vi "Generate Error.vi"(8 "Error In":errorcluster, 10 "Arguments":string[](array[string]), 11 "Error":T1) -> (0 "Error Out":errorcluster)   [LabVIEW 2013, in "LMH-Kodi.lvlib"]
uses:
  LMH-Kodi.lvlib
  Type Defs/Error.ctl
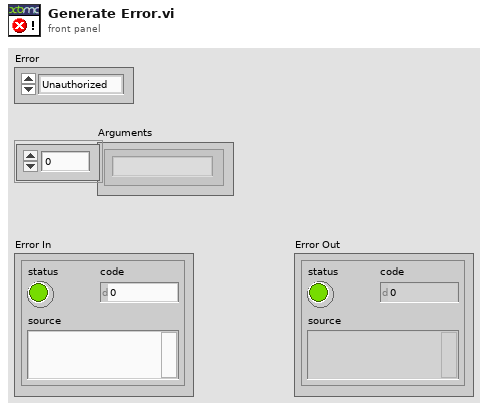
[diagram p1: front panel]
types:
  T1 = typedef "LMH-Kodi.lvlib/Error.ctl" = enum16{"Unauthorized", "XBMC Error", "JSON Parse Error"}
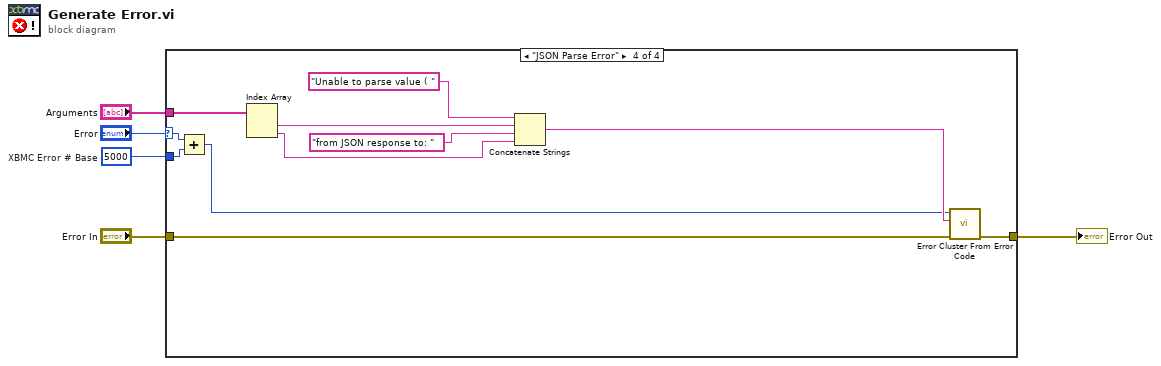
[diagram p0: block diagram]
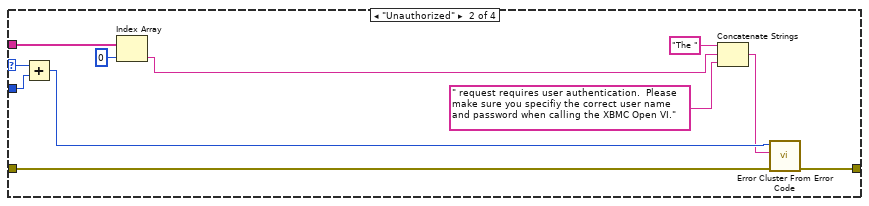
[diagram p3: hidden frame]
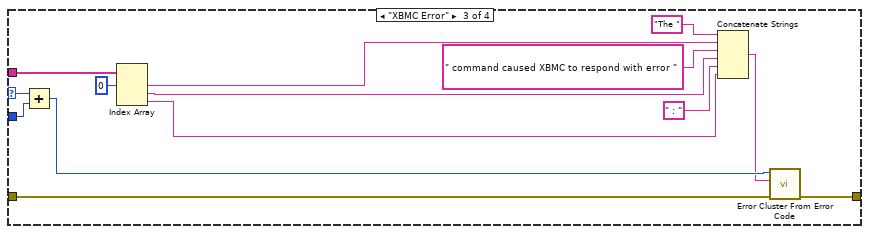
[diagram p4: hidden frame]
diagram:
  w1 = 5000  # XBMC Error # Base
  n1 = case shown="\"JSON Parse Error\"" "Error" {
    selector: "Error" -> [_ w14 w28 w33]
    tunnel: "Error In" -> [w6 w17 w31 w41]
    tunnel: [w6 w16 w30 w42] -> w4
    tunnel: "Arguments" -> [_ w15 w29 w39]
    tunnel: w1 -> [_ w13 w27 w34]
    frame Default {
      # "No Error"
    }
    frame "Unauthorized" {
      n2 = Add(x=w14, y=w13) -> (x+y=w12:i32)
      n3 = Index Array(array=w15, index=0) -> (element=w10:string)
      n4 = Concatenate Strings("The " ("string"), w10, " request requires user authentication.  Please make sure you specifiy the correct user name and password when calling the XBMC Open VI." ("string")) -> (w7:string)
      n5 = call <vilib>:"Error Cluster From Error Code.vi"("error in (no error)"=w17, "error message (\"\")"=w7, "error code (0)"=w12) -> ("error out"=w16:errorcluster)  [unwired: 6 in]
    }
    frame "XBMC Error" {
      n6 = Add(x=w28, y=w27) -> (x+y=w26:i32)
      n7 = Index Array(array=w29, index #1=0 ("index")) -> (element #1=w25:string, element #2=w20:string, element #3=w18:string)  [unwired: 2 in]
      n8 = Concatenate Strings("The " ("string"), w25, " command caused XBMC to respond with error " ("string"), w20, " : " ("string"), w18) -> (w22:string)
      n9 = call <vilib>:"Error Cluster From Error Code.vi"("error in (no error)"=w31, "error message (\"\")"=w22, "error code (0)"=w26) -> ("error out"=w30:errorcluster)  [unwired: 6 in]
    }
    frame "JSON Parse Error" {
      n10 = Add(x=w33, y=w34) -> (x+y=w32:i32)
      n11 = Index Array(array=w39) -> (element #1=w38:string, element #2=w36:string)  [unwired: 2 in]
      n12 = Concatenate Strings("Unable to parse value ( ", w38, "from JSON response to: ", w36) -> (w35:string)
      n13 = call <vilib>:"Error Cluster From Error Code.vi"("error in (no error)"=w41, "error message (\"\")"=w35, "error code (0)"=w32) -> ("error out"=w42:errorcluster)  [unwired: 6 in]
    }
  }
  "Error Out" <- w4
